vi "error_handler.vi"(8 "error in (no error)":errorcluster) -> (0 "error out":errorcluster)   [LabVIEW 2017]
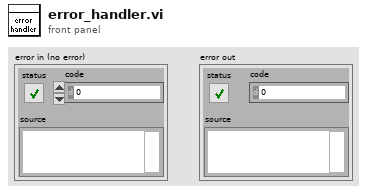
[diagram p1: front panel]
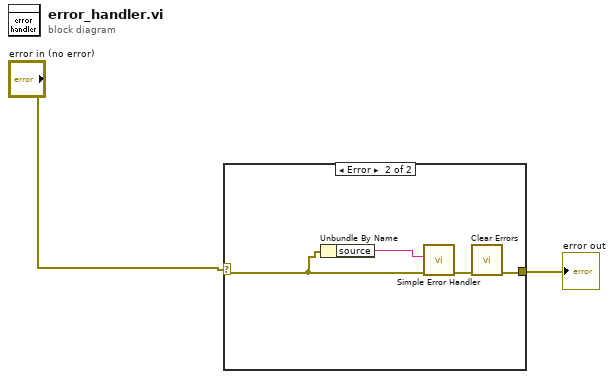
[diagram p0: block diagram]
diagram:
  n1 = case shown="Error" "error in (no error)" {
    selector: "error in (no error)" -> [w3 w5]
    tunnel: [w3 w4] -> w2
    frame No Error {
    }
    frame Error {
      n2 = Unbundle By Name(w5) -> ("source"=w7:string)
      n3 = call <vilib>:"Simple Error Handler.vi"("error source (\" \")"=w7, "error in (no error)"=w5) -> ("error out"=w6:errorcluster)  [unwired: 3 in, 4 out]
      n4 = call <vilib>:"Clear Errors.vi"("error in (no error)"=w6) -> ("error out"=w4:errorcluster)  [unwired: 5 in, 1 out]
    }
  }
  "error out" <- w2
